vi "Get RAM Block.vi"(8 "error in (no error)":errorcluster, 9 "End offset":u64, 10 "Start offset":u64, 11 "RP Instrument in":refnum<class "RP Instrument.lvclass">) -> (0 "error out":errorcluster, 2 "data out":string, 3 "RP Instrument out":refnum<class "RP Instrument.lvclass">)   [LabVIEW 2019, in "RP Instrument.lvclass"]
uses:
  RP Instrument.lvclass
  RP Instrument.lvclass/RP Instrument.ctl
  RP Communicator/RP Communicator.lvclass
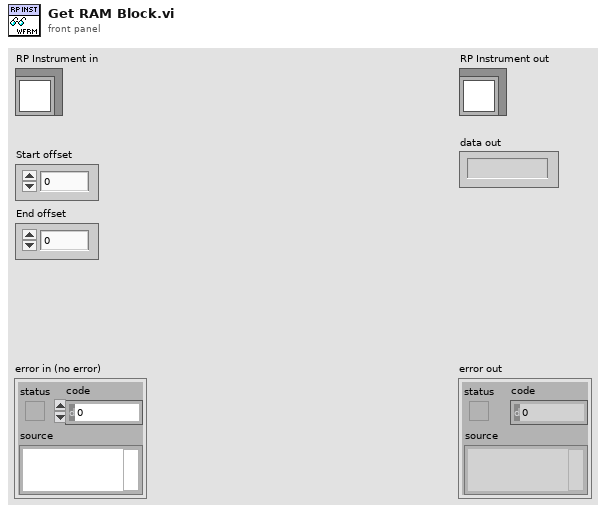
[diagram p1: front panel]
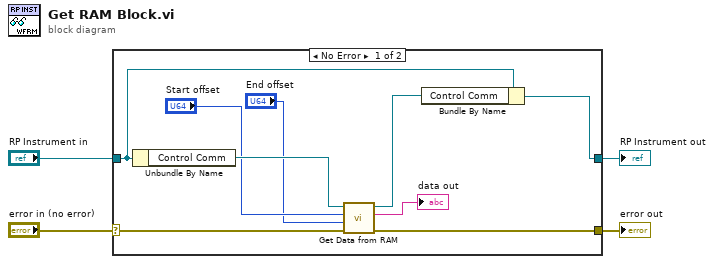
[diagram p0: block diagram]
diagram:
  n1 = case shown="No Error" "error in (no error)" {
    selector: "error in (no error)" -> [w11 w15]
    tunnel: [w8 w15] -> w3
    tunnel: [w10 w14] -> w1
    tunnel: "RP Instrument in" -> [w13 w14]
    frame No Error {
      n2 = Unbundle By Name(w13) -> ("Control Comm"=w12:refnum<class "RP Communicator.lvclass">)
      n3 = call-dynamic "Get Data from RAM.vi"("error in (no error)"=w11, "End offset"="End offset", "Start offset"="Start offset", "RP Communicator in"=w12) -> ("error out"=w8:errorcluster, "data out"=→"data out":string, "RP Communicator out"=w9:refnum<class "RP Communicator.lvclass">)  [unwired: 5 in]
      n4 = Bundle By Name(cluster=w13, "Control Comm"=w9) -> (w10:refnum<class "RP Instrument.lvclass">)
    }
    frame Error {
    }
  }
  "error out" <- w3
  "RP Instrument out" <- w1
